vi "fpga_next_position.vi"(7 "speed":T1, 8 "tip guard position":sgl, 9 "tip guard?":bool, 10 "ready to move?":bool, 11 "target":T1) -> (2 "move completed?":bool, 3 "output":T1)   [LabVIEW 2021]
doc: "Calculate the next position with scan speed.\n\nYou can move only when the scan is active and rady to move status is True."
uses:
  fpga_dtype_sgl_8ch.ctl
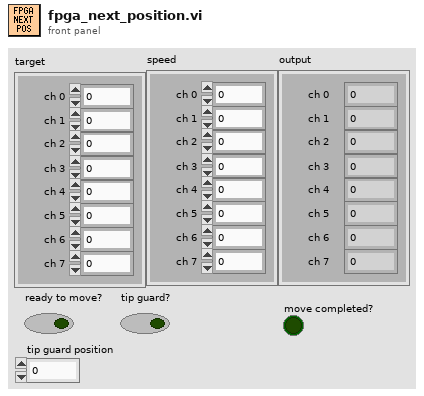
[diagram p1: front panel]
types:
  T1 = typedef "fpga_dtype_sgl_8ch.ctl" = cluster{"ch 0":sgl, "ch 1":sgl, "ch 2":sgl, "ch 3":sgl, "ch 4":sgl, "ch 5":sgl, "ch 6":sgl, "ch 7":sgl}
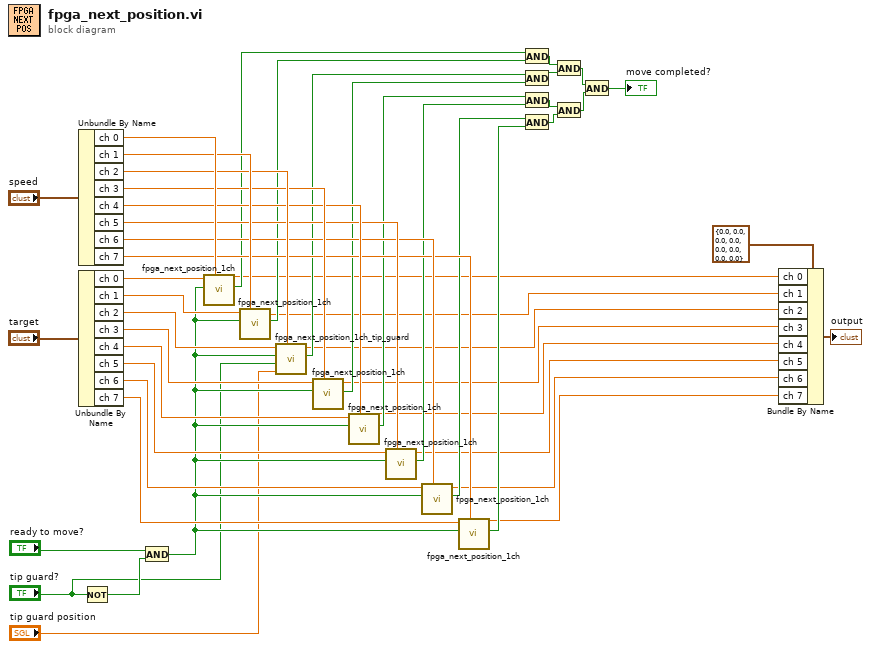
[diagram p0: block diagram]
diagram:
  n1 = Unbundle By Name("speed") -> ("ch 0"=w41:sgl, "ch 1"=w40:sgl, "ch 2"=w39:sgl, "ch 3"=w38:sgl, "ch 4"=w37:sgl, "ch 5"=w36:sgl, "ch 6"=w35:sgl, "ch 7"=w33:sgl)
  n2 = Unbundle By Name("target") -> ("ch 0"=w48:sgl, "ch 1"=w47:sgl, "ch 2"=w46:sgl, "ch 3"=w45:sgl, "ch 4"=w44:sgl, "ch 5"=w43:sgl, "ch 6"=w42:sgl, "ch 7"=w34:sgl)
  n3 = Not(x="tip guard?") -> (.not. x?=w6:bool)
  n4 = And(x="ready to move?", y=w6) -> (x .and. y?=w4:bool)
  n5 = call "fpga_next_position_1ch.vi"("speed"=w41, "ready to move?"=w4, "target"=w48) -> ("move completed?"=w32:bool, "output (out)"=w7:sgl)  [unwired: 7 in]
  n6 = call "fpga_next_position_1ch.vi"("speed"=w40, "ready to move?"=w4, "target"=w47) -> ("move completed?"=w31:bool, "output (out)"=w8:sgl)  [unwired: 7 in]
  n7 = call "fpga_next_position_1ch_tip_guard.vi"("speed"=w39, "Tip guard position"="tip guard position", "tip guard?"="tip guard?", "ready to move?"=w4, "target"=w46) -> ("move completed?"=w30:bool, "output (out)"=w1:sgl)  [unwired: 5 in]
  n8 = call "fpga_next_position_1ch.vi"("speed"=w38, "ready to move?"=w4, "target"=w45) -> ("move completed?"=w29:bool, "output (out)"=w9:sgl)  [unwired: 7 in]
  n9 = call "fpga_next_position_1ch.vi"("speed"=w37, "ready to move?"=w4, "target"=w44) -> ("move completed?"=w28:bool, "output (out)"=w10:sgl)  [unwired: 7 in]
  n10 = call "fpga_next_position_1ch.vi"("speed"=w36, "ready to move?"=w4, "target"=w43) -> ("move completed?"=w27:bool, "output (out)"=w11:sgl)  [unwired: 7 in]
  n11 = call "fpga_next_position_1ch.vi"("speed"=w35, "ready to move?"=w4, "target"=w42) -> ("move completed?"=w26:bool, "output (out)"=w12:sgl)  [unwired: 7 in]
  n12 = call "fpga_next_position_1ch.vi"("speed"=w33, "ready to move?"=w4, "target"=w34) -> ("move completed?"=w25:bool, "output (out)"=w13:sgl)  [unwired: 7 in]
  n13 = And(x=w32, y=w31) -> (x .and. y?=w24:bool)
  n14 = And(x=w30, y=w29) -> (x .and. y?=w23:bool)
  n15 = And(x=w28, y=w27) -> (x .and. y?=w22:bool)
  n16 = And(x=w26, y=w25) -> (x .and. y?=w21:bool)
  n17 = And(x=w24, y=w23) -> (x .and. y?=w19:bool)
  n18 = And(x=w22, y=w21) -> (x .and. y?=w20:bool)
  n19 = And(x=w19, y=w20) -> (x .and. y?=→"move completed?":bool)
  n20 = Bundle By Name(cluster=T1 {"ch 0"=0.0, "ch 1"=0.0, "ch 2"=0.0, "ch 3"=0.0, "ch 4"=0.0, "ch 5"=0.0, "ch 6"=0.0, "ch 7"=0.0} ("sgl 8ch"), "ch 0"=w7, "ch 1"=w8, "ch 2"=w1, "ch 3"=w9, "ch 4"=w10, "ch 5"=w11, "ch 6"=w12, "ch 7"=w13) -> (→"output":T1)
